vi "Fire LogStateChanged Event_DAQ.vi"(6 "bypass (F)":bool, 8 "error in (no error)":errorcluster, 10 "DAQState":variant, 11 "Log_Engine in":refnum<class "Log_Engine.lvclass">) -> (0 "error out":errorcluster, 3 "Log_Engine out":refnum<class "Log_Engine.lvclass">)   [LabVIEW 2019, in "Log_Engine.lvclass"]
doc: "Developed by Kevin Thompson\nkevin@thompsonengineering.net\n\nCopyright 2018-2020\nThompson Engineering, LLC"
uses:
  Log_Engine.lvclass
  Common/DataTypes/LogState--enum.ctl
  DataTypes/LogStateChg EvData--cluster.ctl
  DataTypes/LogStateEvData--cluster.ctl
  Log_Engine.lvclass/Log_Engine.ctl
  Accessors/Get PublicEvents.vi
  Accessors/Get LogState.vi
  Accessors/Set LogState.vi
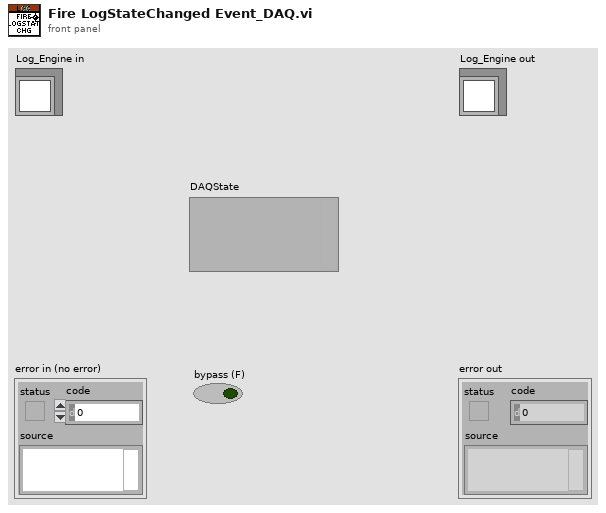
[diagram p1: front panel]
types:
  T1 = typedef "Log_Engine.lvclass/LogStateChg EvData--cluster.ctl" = cluster{"Time Stamp":timestamp, "OLD State":T2, "NEW State":T2}
  T2 = typedef "Log_Engine.lvclass/LogStateEvData--cluster.ctl" = cluster{"LogState":T3, "vData":variant}
  T3 = typedef "LogState--enum.ctl" = enum16{"Unknown", "Stopped", "Running", "Error"}
  T4 = typedef "Log_Engine.lvclass/Public Events--cluster.ctl" = cluster{"Log_Engine.AsyncCmd Event":refnum<user-event>, "Log_Engine.AsyncMsg Event":refnum<user-event>, "stop process":refnum<user-event>, "Log_Engine.LogStateChg Ev":refnum<user-event>, "Log_Engine.TDMSStateChg Ev":refnum<user-event>}
  T5 = typedef "Type Descriptor Enumeration__ogtk.ctl" = enum8{"<Null>", "I8", "I16", "I32", "I64", "U8", "U16", "U32", "U64", "SGL", "DBL", "EXT", "CSG", "CDB", "CXT", "0x0F", "0x10", "0x11", "0x12", "0x13", "0x14", "Enum U8", "Enum U16", "Enum U32", "Enum U64", "SGL PQ", "DBL PQ", "EXT PQ", "CSG PQ", "CDB PQ", "CXT PQ", "0x1F", "0x20", "Boolean", "0x22", "0x23", "0x24", "0x25", "0x26", "0x27", "0x28", "0x29", "0x2A", "0x2B", "0x2C", "0x2D", "0x2E", "0x2F", "String", "0x31", "Path", "Pict", "0x34", "0x35", "0x36", "DAQ", "0x38", "0x39", "0x3A", "0x3B", "0x3C", "0x3D", "0x3E", "0x3F", "Array", "0x41", "0x42", "0x43", "0x44", "0x45", "0x46", "0x47", "0x48", "0x49", "0x4A", "0x4B", "0x4C", "0x4D", "0x4E", "0x4F", "Cluster", "0x51", "0x52", "Variant", "Waveform", "0x55", "0x56", "0x57", "0x58", "0x59", "0x5A", "0x5B", "0x5C", "0x5D", "0x5E", "0x5F", "0x60", "0x61", "0x62", "0x63", "0x64", "0x65", "0x66", "0x67", "0x68", "0x69", "0x6A", "0x6B", "0x6C", "0x6D", "0x6E", "0x6F", "Refnum"}
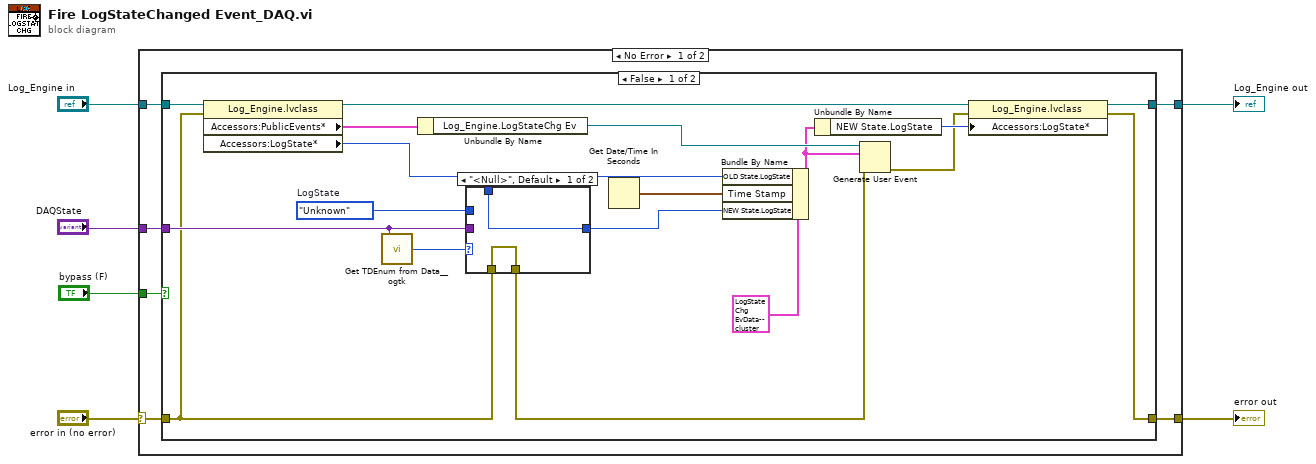
[diagram p0: block diagram]
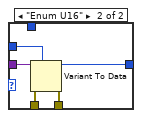
[diagram p2: hidden frame]
diagram:
  n1 = case shown="No Error" "error in (no error)" {
    selector: "error in (no error)" -> [w8 w41]
    tunnel: [w9 w41] -> w5
    tunnel: [w10 w40] -> w3
    tunnel: "Log_Engine in" -> [w12 w40]
    tunnel: "DAQState" -> [w11 _]
    tunnel: "bypass (F)" -> [w7 _]
    frame No Error {
      n2 = case shown="False" w7 {
        tunnel: w12 -> [w29 w39]
        tunnel: w11 -> [w27 _]
        tunnel: [w24 w39] -> w10
        tunnel: [w21 w38] -> w9
        tunnel: w8 -> [w20 w38]
        frame False {
          w15 = LogState--enum."Unknown"  # LogState
          n3 = property class="Log_Engine.lvclass"(reference=w29, error in=w20) -> (reference out=w17:refnum<class "Log_Engine.lvclass">, "Accessors:PublicEvents*"=w18:T4, "Accessors:LogState*"=w16:T3)  [unwired: 1 out]
          n4 = call <userlib>:"Get TDEnum from Data__ogtk.vi"("Data"=w27) -> ("Type Descriptor Enumeration"=w28:T5)  [unwired: 4 in]
          n5 = Unbundle By Name(w18) -> ("Log_Engine.LogStateChg Ev"=w19:refnum<user-event>)
          n6 = case shown="\"<Null>\", Default" w28 {
            tunnel: w16 -> [w31 _]
            tunnel: w27 -> [_ w37]
            tunnel: [w31 w36] -> w26
            tunnel: w15 -> [_ w35]
            tunnel: w20 -> [w32 w34]
            tunnel: [w32 w33] -> w25
            frame "<Null>", Default {
            }
            frame "Enum U16" {
              n7 = Variant To Data(error in=w34, type=w35, Variant=w37) -> (data=w36:T3, error out=w33:errorcluster)
            }
          }
          n8 = Get Date/Time In Seconds() -> (seconds since 1Jan1904=w30:timestamp)
          n9 = Bundle By Name(cluster=T1 {"Time Stamp"=timestamp(0 s since 1904-01-01), "OLD State"={"LogState"=enum."Unknown", "vData"=variant}, "NEW State"={"LogState"=enum."Unknown", "vData"=variant}} ("LogStateChg EvData"), "OLD State.LogState"=w16, "Time Stamp"=w30, "NEW State.LogState"=w26) -> (w13:T1)
          n10 = Unbundle By Name(w13) -> ("NEW State.LogState"=w23:T3)
          n11 = Generate User Event(user event=w19, event data cluster=w13, error in=w25) -> (error out=w22:errorcluster)  [unwired: 1 in, 1 out]
          n12 = property class="Log_Engine.lvclass"(reference=w17, error in=w22, "Accessors:LogState*"=w23) -> (reference out=w24:refnum<class "Log_Engine.lvclass">, error out=w21:errorcluster)
        }
        frame True {
        }
      }
    }
    frame Error {
    }
  }
  "error out" <- w5
  "Log_Engine out" <- w3
